vi "UEGO card.vi"(8 "error in (no error)":errorcluster, 11 "Node Ptr":T3 format="%.0x") -> (0 "error out":errorcluster)   [LabVIEW 2014, in "SLSC configuration System Explorer.lvlib"]
uses:
  SLSC configuration System Explorer.lvlib
  <vilib>/NI Veristand/Custom Device API/Custom Device Item Ref.ctl
  Type Defs/Card Position.ctl
  Shared/SPI Utility/Slot #.ctl
  Shared/Constants.vi
  <vilib>/NI Veristand/Custom Device API/Get Item Property (U32).vi
  <vilib>/NI Veristand/Custom Device API/Get Item Property (String).vi
  <vilib>/NI Veristand/Custom Device API/Set Item Property (U32).vi
  <vilib>/NI Veristand/Custom Device API/Custom Device API.lvlib
  Shared/SLSC configuration Shared.lvlib
panel:
  out "FPGA Item Name":string
  in  "Header 3":cluster{"Section Name":string}={"Section Name"="Oxygen Sensor Simulation Card Settings"}
  in  "Header 2":cluster{"Section Name":string}={"Section Name"="Oxygen Sensor Simulation Card Settings"}
  in  "Calibration Time (µsec)":u32
  in  "Hardware Settling Time (µsec)":u32
  in  "Card Position":T1 {"Slot #" max=15}
  in  "Header":cluster{"Section Name":string}={"Section Name"="Oxygen Sensor Simulation Card Settings"}
  in  "Description":string
  in  "Name":string
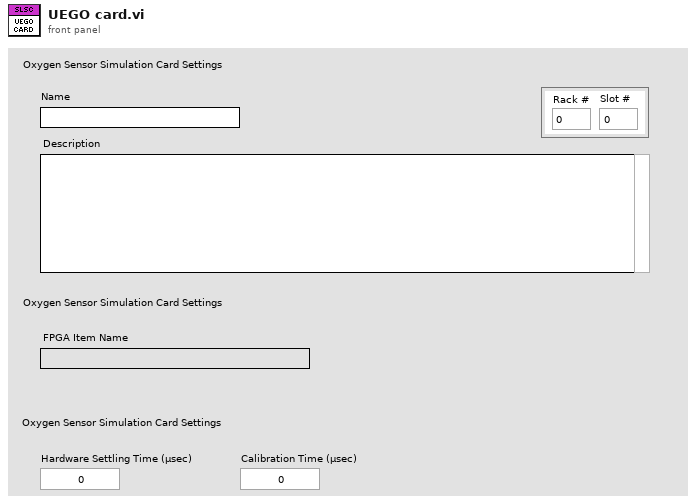
[diagram p1: front panel]
types:
  T1 = typedef "SLSC configuration Shared.lvlib/Card Position.ctl" = cluster{"Rack #":u8, "Slot #":T2}
  T2 = typedef "SLSC configuration Shared.lvlib/Slot #.ctl" = u8
  T3 = typedef "Custom Device API.lvlib/Custom Device Item Ref.ctl" = u64
  T4 = typedef "Custom Device API.lvlib/Custom Device Commands.ctl" = enum16{"Default", "Item renamed", "Shutdown", "Dynamic button pressed"}
  T5 = typedef "Custom Device API.lvlib/Custom Device Item Info.ctl" = cluster{"Name":string, "Is Channel":bool, "GUID":string, "Is Waveform":bool}
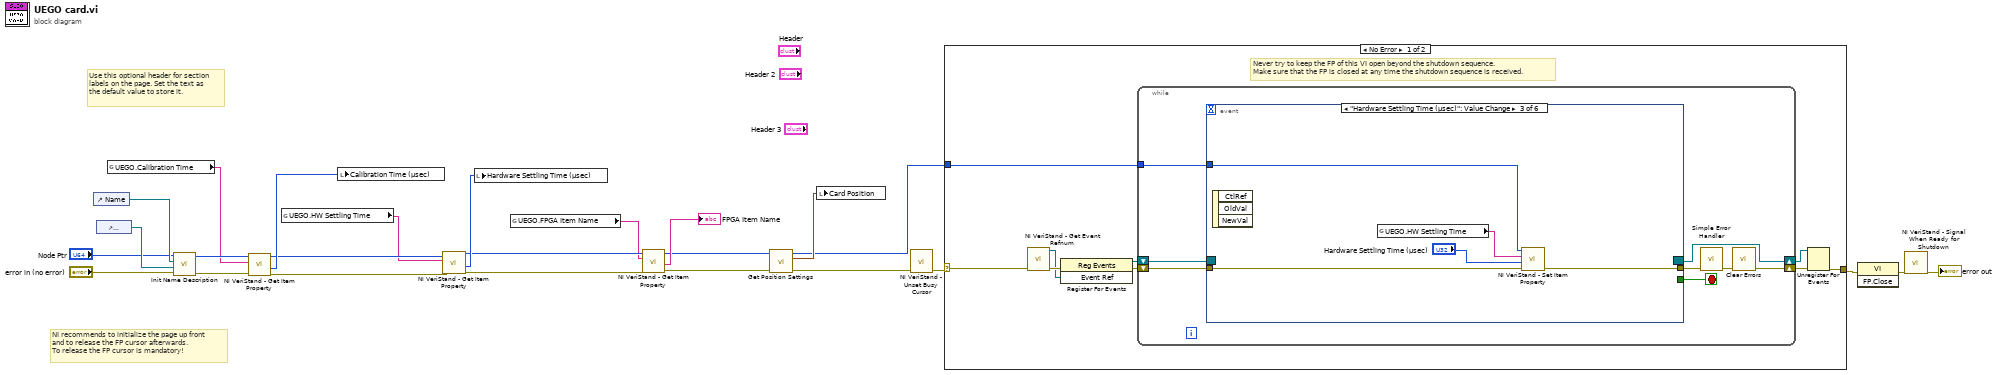
[diagram p0: block diagram]
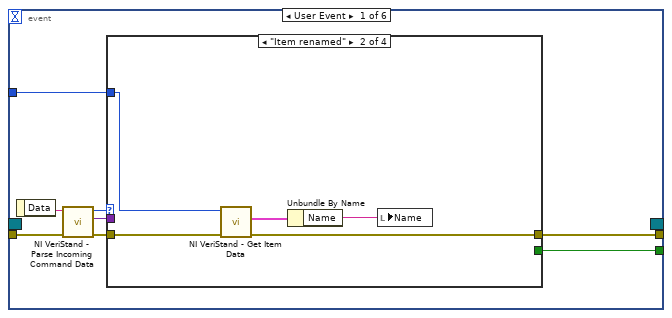
[diagram p2: hidden frame]
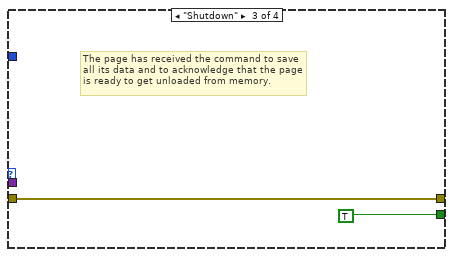
[diagram p4: hidden frame]
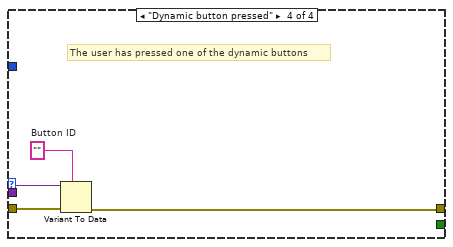
[diagram p5: hidden frame]
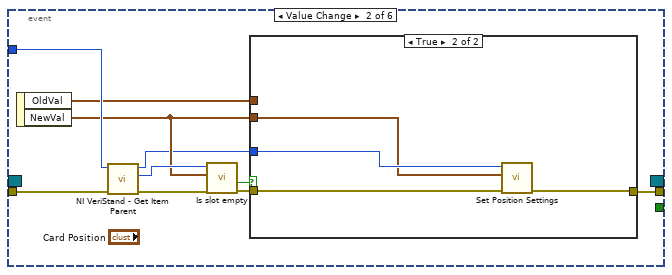
[diagram p6: hidden frame]
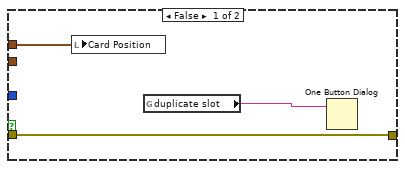
[diagram p7: hidden frame]
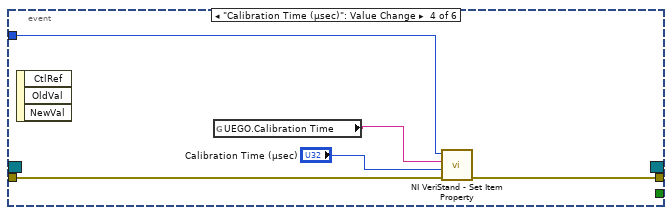
[diagram p8: hidden frame]
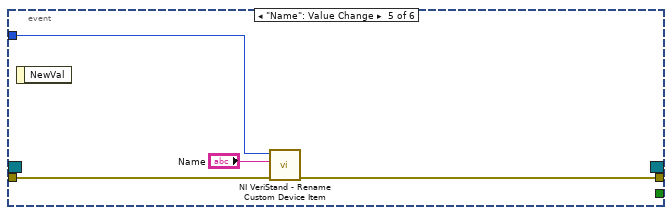
[diagram p9: hidden frame]
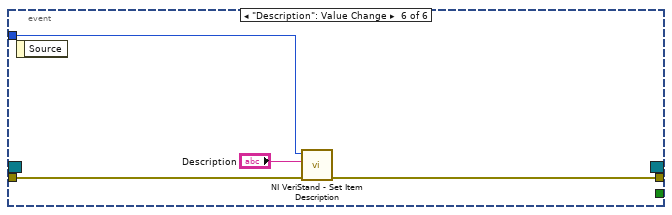
[diagram p10: hidden frame]
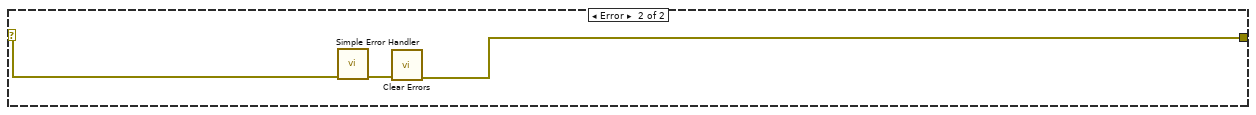
[diagram p11: hidden frame]
diagram:
  # "Use this optional header for section labels on the page. Set the text as the default value to store it."
  # "NI recommends to initialize the page up front\nand to release the FP cursor afterwards.\nTo release the FP cursor is mandatory!"
  n1 = control-ref of="Name"() -> (w21:refnum<vi>)
  n2 = control-ref of="Description"() -> (w20:refnum<vi>)
  n3 = global read "Constants.vi" "UEGO.Calibration Time"() -> (w12:string)
  n4 = call "Init Name Description.vi"("error in (no error)"="error in (no error)", "Description"=w20, "Name"=w21, "Node Ptr"="Node Ptr") -> ("error out"=w14:errorcluster, "Node Ptr out"=w13:T3)  [unwired: 6 in]
  n5 = call-poly <vilib>:"NI VeriStand - Get Item Property.vi"("error in (no error)"=w14, "Property Name"=w12, "Item Ref in"=w13) -> ("error out"=w10:errorcluster, "Value"=w11:u32, "Item Ref out"=w9:T3)  [unwired: 5 in, 1 out]
  n6 = global read "Constants.vi" "UEGO.HW Settling Time"() -> (w8:string)
  n7 = local write "Calibration Time (µsec)"(w11) -> ()
  n8 = call-poly <vilib>:"NI VeriStand - Get Item Property.vi"("error in (no error)"=w10, "Property Name"=w8, "Item Ref in"=w9) -> ("error out"=w6:errorcluster, "Value"=w7:u32, "Item Ref out"=w5:T3)  [unwired: 5 in, 1 out]
  n9 = local write "Hardware Settling Time (µsec)"(w7) -> ()
  n10 = global read "Constants.vi" "UEGO.FPGA Item Name"() -> (w4:string)
  n11 = call-poly <vilib>:"NI VeriStand - Get Item Property.vi"("error in (no error)"=w6, "Property Name"=w4, "Item Ref in"=w5) -> ("error out"=w1:errorcluster, "Value"=→"FPGA Item Name":string, "Item Ref out"=w2:T3)  [unwired: 5 in, 1 out]
  n12 = call "Get Position Settings.vi"("error in (no error)"=w1, "Item Ref in"=w2) -> ("error out"=w16:errorcluster, "Card Position"=w17:T1, "Item Ref out"=w15:T3)  [unwired: 7 in]
  n13 = local write "Card Position"(w17) -> ()
  n14 = call <vilib>:"NI VeriStand - Unset Busy Cursor.vi"("error in (no error)"=w16) -> ("error out"=w22:errorcluster)  [unwired: 10 out]
  n15 = case shown="No Error" w22 {
    selector: w22 -> [w27 w100]
    tunnel: [w31 w98] -> w25
    tunnel: w15 -> [w26 _]
    frame No Error {
      # "Never try to keep the FP of this VI open beyond the shutdown sequence.\nMake sure that the FP is closed at any time the shutdown sequence is received."
      n16 = call <vilib>:"NI VeriStand - Get Event Refnum.vi"("error in (no error)"=w27) -> ("error out"=w34:errorcluster, "Event Ref"=w30:refnum<user-event>)  [unwired: 9 out]
      n17 = register-events(error in=w34, w30) -> (reference out=w28:refnum<event-registration>, error out=w29:errorcluster)  [unwired: 1 in]
      n18 = while {
        shift-right: [w36] -> w32
        shift-left: w29 -> [w41]
        shift-right: [w42] -> w33
        shift-left: w28 -> [w40]
        tunnel: w26 -> [w35]
        stop <- w39 stop-if-true
        n19 = event shown="[2] \"Hardware Settling Time (µsec)\": Value Change" {
          selector: w40 -> [_ _ _ _ _ _]
          dyn-events: [_ _ _ _ _ _] -> w42
          timeout: _ -> [_ _ _ _ _ _]
          tunnel: w41 -> [w50 w71 w84 w89 w93 w97]
          tunnel: [w46 _ _ _ _ _] -> w39
          tunnel: [w45 w72 w83 w88 w92 w96] -> w38
          tunnel: w35 -> [w43 w70 w81 w87 w90 w94]
          event User Event {
            n20 = event-data() -> ("Data"=w49:string)  [unwired: 1 out]
            n21 = call <vilib>:"NI VeriStand - Parse Incoming Command Data.vi"("error in (no error)"=w50, "Incoming data"=w49) -> ("error out"=w48:errorcluster, "Outgoing data"=w44:variant, "Action"=w47:T4)  [unwired: 7 out]
            n22 = case shown="\"Item renamed\"" w47 {
              tunnel: w48 -> [w51 w56 w57 w62]
              tunnel: [_ _ TRUE _] -> w46
              tunnel: [w51 w54 w57 w59] -> w45
              tunnel: w44 -> [_ _ _ w61]
              tunnel: w43 -> [_ w52 _ _]
              frame "Default", Default {
              }
              frame "Item renamed" {
                n23 = call <vilib>:"NI VeriStand - Get Item Data.vi"("error in (no error)"=w56, "Item Ref in"=w52) -> ("error out"=w54:errorcluster, "Item Info"=w55:T5)  [unwired: 8 out]
                n24 = Unbundle By Name(w55) -> ("Name"=w53:string)
                n25 = local write "Name"(w53) -> ()
              }
              frame "Shutdown" {
                # "The page has received the command to save all its data and to acknowledge that the page is ready to get unloaded from memory."
              }
              frame "Dynamic button pressed" {
                w60 = ""  # Button ID
                # "The user has pressed one of the dynamic buttons"
                n26 = Variant To Data(error in=w62, type=w60, Variant=w61) -> (error out=w59:errorcluster)  [unwired: 1 out]
              }
            }
          }
          event Value Change {
            n27 = event-data() -> ("OldVal"=w63:T1, "NewVal"=w65:T1)  [unwired: 1 out]
            n28 = call <vilib>:"NI VeriStand - Get Item Parent.vi"("error in (no error)"=w71, "Item Ref in"=w70) -> ("error out"=w69:errorcluster, "Parent Ref"=w68:T3, "Item Ref out"=w64:T3)  [unwired: 6 in, 1 out]
            n29 = call "Is slot empty.vi"("error in (no error)"=w69, "Card Position"=w65, "Devcie Ref in"=w68) -> ("error out"=w66:errorcluster, "Empty?"=w67:bool)  [unwired: 6 in, 1 out]
            n30 = case shown="True" w67 {
              tunnel: [w75 w76] -> w72
              tunnel: w66 -> [w75 w79]
              tunnel: w65 -> [_ w77]
              tunnel: w64 -> [_ w78]
              tunnel: w63 -> [w73 _]
              frame False {
                n31 = local write "Card Position"(w73) -> ()
                n32 = global read "Constants.vi" "duplicate slot"() -> (w74:string)
                n33 = One Button Dialog(message=w74) -> ()  [unwired: 1 in, 1 out]
              }
              frame True {
                n34 = call "Set Position Settings.vi"("error in (no error)"=w79, "Card Position"=w77, "Item Ref in"=w78) -> ("error out"=w76:errorcluster)  [unwired: 7 in, 1 out]
              }
            }
          }
          event "Hardware Settling Time (µsec)": Value Change {
            n35 = event-data() -> ()  [unwired: 4 out]
            n36 = global read "Constants.vi" "UEGO.HW Settling Time"() -> (w80:string)
            n37 = call-poly <vilib>:"NI VeriStand - Set Item Property.vi"("error in (no error)"=w84, "Value"="Hardware Settling Time (µsec)", "Property Name"=w80, "Item Ref in"=w81) -> ("error out"=w83:errorcluster)  [unwired: 5 in, 2 out]
          }
          event "Calibration Time (µsec)": Value Change {
            n38 = event-data() -> ()  [unwired: 4 out]
            n39 = global read "Constants.vi" "UEGO.Calibration Time"() -> (w85:string)
            n40 = call-poly <vilib>:"NI VeriStand - Set Item Property.vi"("error in (no error)"=w89, "Value"="Calibration Time (µsec)", "Property Name"=w85, "Item Ref in"=w87) -> ("error out"=w88:errorcluster)  [unwired: 5 in, 2 out]
          }
          event "Name": Value Change {
            n41 = event-data() -> ()  [unwired: 2 out]
            n42 = call <vilib>:"NI VeriStand - Rename Custom Device Item.vi"("error in (no error)"=w93, "New Name"="Name", "Item Ref in"=w90) -> ("error out"=w92:errorcluster)  [unwired: 1 in, 7 out]
          }
          event "Description": Value Change {
            n43 = event-data() -> ()  [unwired: 2 out]
            n44 = call <vilib>:"NI VeriStand - Set Item Description.vi"("error in (no error)"=w97, "Description"="Description", "Item Ref in"=w94) -> ("error out"=w96:errorcluster)  [unwired: 8 out]
          }
        }
        n45 = call <vilib>:"Simple Error Handler.vi"("error in (no error)"=w38) -> ("error out"=w37:errorcluster)  [unwired: 1 in, 7 out]
        n46 = call <vilib>:"Clear Errors.vi"("error in (no error)"=w37) -> ("error out"=w36:errorcluster)  [unwired: 1 in, 5 out]
      }
      n47 = Unregister For Events(event registration refnum=w33, error in=w32) -> (error out=w31:errorcluster)
    }
    frame Error {
      n48 = call <vilib>:"Simple Error Handler.vi"("error in (no error)"=w100) -> ("error out"=w99:errorcluster)  [unwired: 1 in, 7 out]
      n49 = call <vilib>:"Clear Errors.vi"("error in (no error)"=w99) -> ("error out"=w98:errorcluster)  [unwired: 1 in, 5 out]
    }
  }
  n50 = invoke class="VI" method="FP.Close"(error in=w25) -> (error out=w24:errorcluster)  [unwired: 2 in, 2 out]
  n51 = call <vilib>:"NI VeriStand - Signal When Ready for Shutdown.vi"("error in (no error)"=w24) -> ("error out"=→"error out":errorcluster)  [unwired: 10 out]
